vi "Test_DMM 34461A.vi"() -> ()   [LabVIEW 2018]
uses:
  Sct_Cmd.ctl
panel:
  out "Measurement":dbl format="%#.10f"
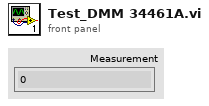
[diagram p1: front panel]
types:
  T1 = enum16{"100μA", "1mA", "10mA", "100mA", "1A", "3A", "10A"}
  T2 = typedef "Sct_Cmd.ctl" = enum16{"Init", "Setting", "1SampleRead", "MultiSampleRead", "Close"}
  T3 = cluster{"Auto Range":bool, "Manual Range (1)":dbl, "Absolute Resolution (1E-6)":dbl}
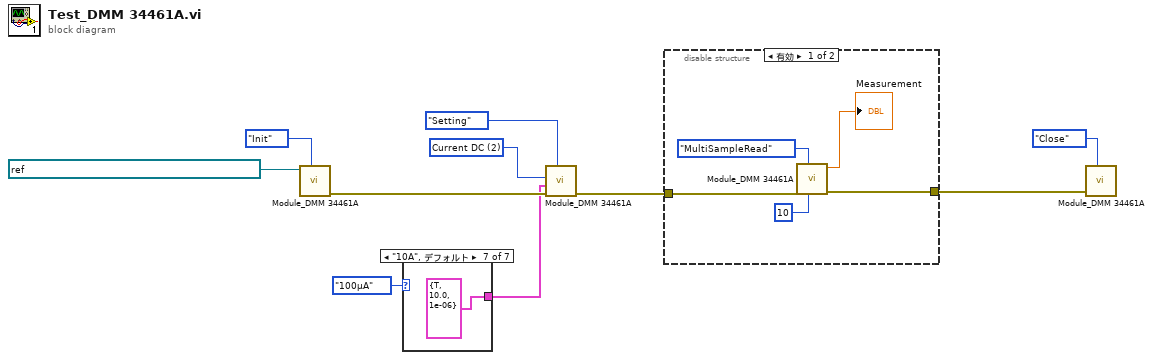
[diagram p0: block diagram]
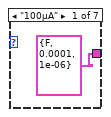
[diagram p2: hidden frame]
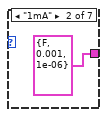
[diagram p3: hidden frame]
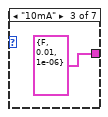
[diagram p4: hidden frame]
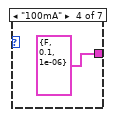
[diagram p5: hidden frame]
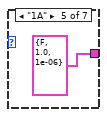
[diagram p6: hidden frame]
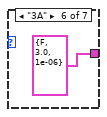
[diagram p7: hidden frame]
diagram:
  w4 = 2 items=["Continuity", "Current AC", "Current DC", "Diode", "Frequency", "Resistance 4-wire", "Period", "Resistance 2-wire", "Temperature", "Voltage AC", "Voltage DC", "Voltage DC Ratio"] ("Measurement Function")
  n1 = call "Module_DMM 34461A.vi"("Sct_Cmd"=Sct_Cmd."Init", "VISA resource name"=refnum<visa-resource-name> "USB0::0x2A8D::0x1301::MY57215744::INSTR") -> ("error out"=w6:errorcluster)  [unwired: 8 in, 1 out]
  n2 = case shown="\"10A\", デフォルト" T1."100μA" ("レンジ") {
    tunnel: [T3 {"Auto Range"=FALSE, "Manual Range (1)"=0.0001, "Absolute Resolution (1E-6)"=1e-06} ("Range") T3 {"Auto Range"=FALSE, "Manual Range (1)"=0.001, "Absolute Resolution (1E-6)"=1e-06} ("Range") T3 {"Auto Range"=FALSE, "Manual Range (1)"=0.01, "Absolute Resolution (1E-6)"=1e-06} ("Range") T3 {"Auto Range"=FALSE, "Manual Range (1)"=0.1, "Absolute Resolution (1E-6)"=1e-06} ("Range") T3 {"Auto Range"=FALSE, "Manual Range (1)"=1.0, "Absolute Resolution (1E-6)"=1e-06} ("Range") T3 {"Auto Range"=FALSE, "Manual Range (1)"=3.0, "Absolute Resolution (1E-6)"=1e-06} ("Range") T3 {"Auto Range"=TRUE, "Manual Range (1)"=10.0, "Absolute Resolution (1E-6)"=1e-06} ("Range")] -> w1
    frame "100μA" {
    }
    frame "1mA" {
    }
    frame "10mA" {
    }
    frame "100mA" {
    }
    frame "1A" {
    }
    frame "3A" {
    }
    frame "10A", Default {
    }
  }
  n3 = call "Module_DMM 34461A.vi"("Sct_Cmd"=Sct_Cmd."Setting", "error in (no error)"=w6, "Range"=w1, "Measurement Function"=w4) -> ("error out"=w5:errorcluster)  [unwired: 6 in, 1 out]
  n4 = disable-structure shown="有効" {
    disable-tunnel: [w20 _] -> w9
    disable-tunnel: w5 -> [w18 _]
    frame Enabled {
      n5 = call "Module_DMM 34461A.vi"("Sample Count"=10, "Sct_Cmd"=Sct_Cmd."MultiSampleRead", "error in (no error)"=w18) -> ("error out"=w20:errorcluster, "Measurement"=→"Measurement":dbl)  [unwired: 7 in]
    }
    frame Disabled {
    }
  }
  n6 = call "Module_DMM 34461A.vi"("Sct_Cmd"=Sct_Cmd."Close", "error in (no error)"=w9) -> ()  [unwired: 8 in, 2 out]
